vi "Stop-Process1.vi"(8 "error in (no error)":errorcluster, 11 "Object ref in":T1) -> (0 "error out":errorcluster, 3 "Object ref out":T1)   [LabVIEW 2013, in "HardwareCharacterization.lvlib" / "HC-Main.lvclass"]
uses:
  HC-Main.lvclass
  Object-reference.ctl
  HC-Main.lvclass/HC-Main.ctl
  Read SM1000.vi
  SM1000/HC-SM1000.lvclass
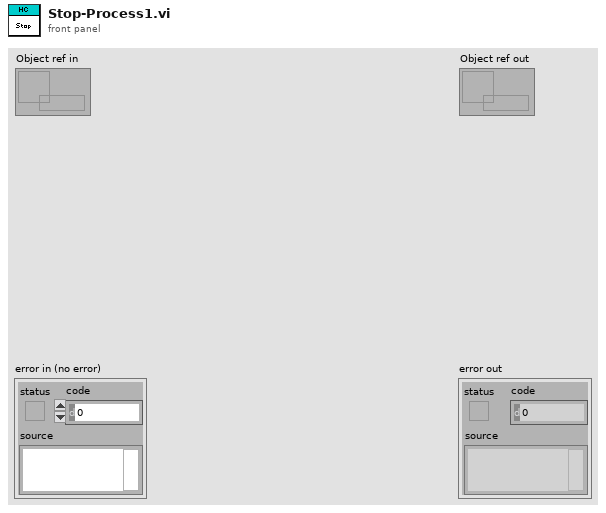
[diagram p1: front panel]
types:
  T1 = typedef "HardwareCharacterization.lvlib/HC-Main.lvclass/Object-reference.ctl" = refnum<data-value>
  T2 = typedef "HardwareCharacterization.lvlib/HC-SM1000.lvclass/Object-reference.ctl" = refnum<data-value>
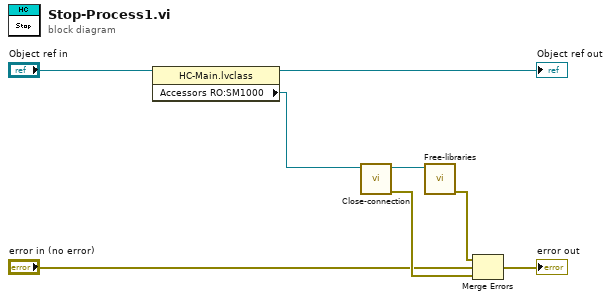
[diagram p0: block diagram]
diagram:
  n1 = property class="HC-Main.lvclass"(reference="Object ref in") -> (reference out=→"Object ref out":T1, "Accessors RO:SM1000"=w6:T2)  [unwired: 1 in, 1 out]
  n2 = call "Close-connection.vi"("SM1000-control in"=w6) -> ("error out"=w3:errorcluster, "SM1000-control out"=w1:T2)  [unwired: 8 in, 1 out]
  n3 = call "Free-libraries.vi"("SM1000-control in"=w1) -> ("error out"=w5:errorcluster)  [unwired: 8 in, 2 out]
  n4 = Merge Errors(w5, "error in (no error)", w3) -> (→"error out":errorcluster)
